vi "sendPriorityData.vi"(8 "error in (no error)":errorcluster, 9 "Additional content":string, 10 "Priority message":T1=enum."SetOffset", 11 "SM1000-control in":T2) -> (0 "error out":errorcluster, 3 "SM1000-control out":T2)   [LabVIEW 2013, in "SLMControl.lvlib" / "SM1000.lvclass"]
doc: "Send priority data to an EC device session.\n\nAn independent and parallel communication channel is provided to the controller to pass \"out-of-band\" commands. This channel of communication is used to send urgent commands to the controller, such as an abort message, or pause/resume messages.\nThe method returns as soon as the message is sent, not when the operation is actually performed on the target. Some messages, however, create response events when the action is completed, such as \"Abort\" or \"GetRegisters\"."
uses:
  SM1000.lvclass
  Object-reference.ctl
  Priority-messages.ctl
  SM1000.lvclass/SM1000.ctl
  Custom-errors.ctl
  C:/Users/vangeste/Desktop/2015-06-02 - SLM - MAIF/HC-HardwareCharacterization/Sources/SM1000/LECSession.dll
  HC-HardwareCharacterization/Sources/SM1000/LECSession.dll
  DOTNET-error-int.vi
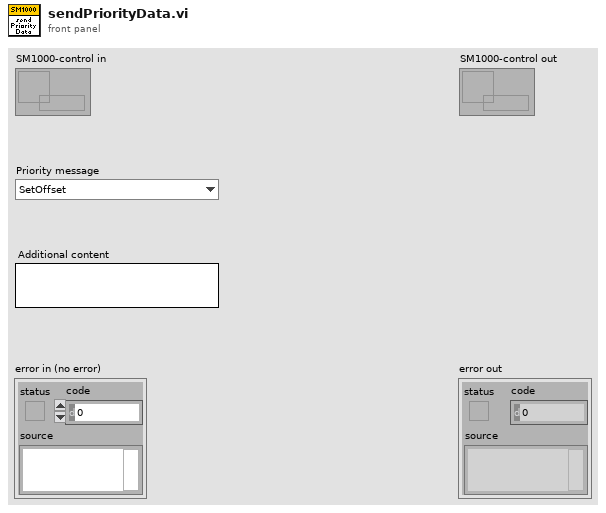
[diagram p1: front panel]
types:
  T1 = typedef "SLMControl.lvlib/SM1000.lvclass/Priority-messages.ctl" = enum16{"Abort", "Restart", "Suspend", "Resume", "GetRegisters", "SetInterlockEnable", "SetOffset"}
  T2 = typedef "SLMControl.lvlib/SM1000.lvclass/Object-reference.ctl" = refnum<data-value>
  T3 = typedef "SLMControl.lvlib/SM1000.lvclass/Custom-errors.ctl" = enum16{"No error", "Not implemented", "Command not recognized", "Invalid input", "No connection", "Timeout", "Resource not loaded"}
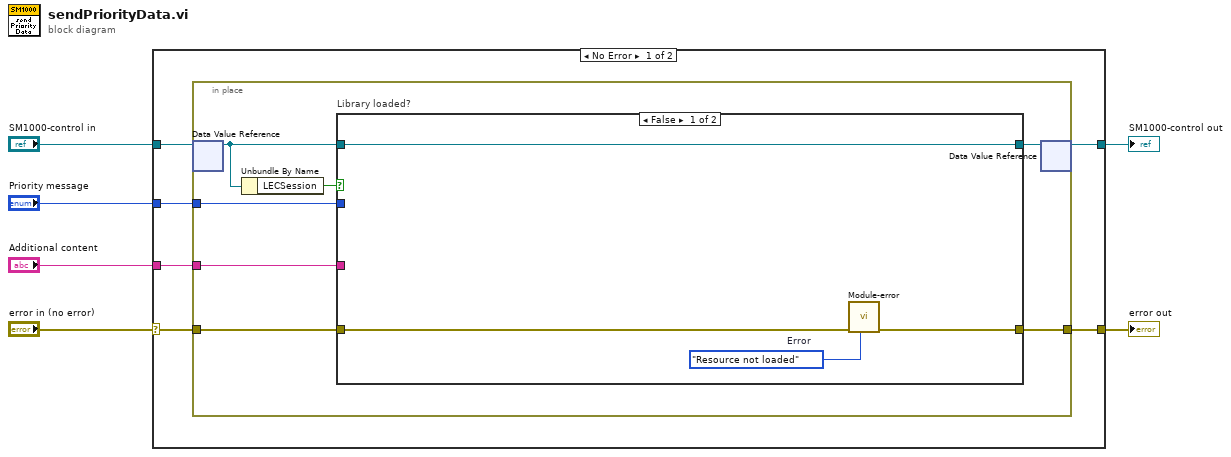
[diagram p0: block diagram]
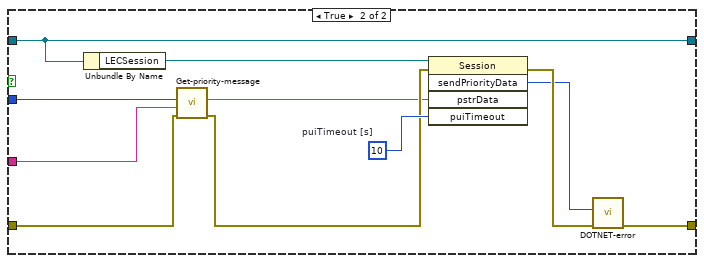
[diagram p2: hidden frame]
diagram:
  n1 = case shown="No Error" "error in (no error)" {
    selector: "error in (no error)" -> [w10 w36]
    tunnel: [w9 w36] -> w5
    tunnel: [w11 w35] -> w3
    tunnel: "SM1000-control in" -> [w12 w35]
    tunnel: "Priority message" -> [w8 _]
    tunnel: "Additional content" -> [w7 _]
    frame No Error {
      n2 = in-place {
        in-place-border: w10 -> [w19]
        in-place-border: [w16] -> w9
        in-place-border: w8 -> [w14]
        in-place-border: w7 -> [w13]
        n3 = in-place-dvr #1(w12) -> (w17:refnum<class "SM1000.lvclass">)  [unwired: 1 out]
        n4 = Unbundle By Name(w17) -> ("LECSession"=w18:bool)
        n5 = case "Library loaded?" shown="False" w18 {
          tunnel: w19 -> [w23 w29]
          tunnel: w17 -> [w21 w33]
          tunnel: [w22 w26] -> w16
          tunnel: [w21 w33] -> w15
          tunnel: w14 -> [_ w31]
          tunnel: w13 -> [_ w30]
          frame False {
            w20 = Custom-errors."Resource not loaded"  # Error
            n6 = call "Module-error.vi"("Error"=w20, "error in (no error)"=w23) -> ("error out"=w22:errorcluster)  [unwired: 9 in]
          }
          frame True {
            w32 = u32 10  # puiTimeout [s]
            n7 = Unbundle By Name(w33) -> ("LECSession"=w34:refnum<k24>)
            n8 = call "Get-priority-message.vi"("error in (no error)"=w29, "Additional content"=w30, "Priority message"=w31) -> ("error out"=w28:errorcluster, "Message string"=w27:string)  [unwired: 7 in]
            n9 = invoke class="Session" method="sendPriorityData"(reference=w34, error in=w28, "pstrData"=w27, "puiTimeout"=w32) -> (error out=w25:errorcluster, "sendPriorityData"=w24:u32)  [unwired: 1 in, 3 out]
            n10 = call-poly "DOTNET-error.vi"("error in (no error)"=w25, "Retun code"=w24) -> ("error out"=w26:errorcluster)  [unwired: 9 in]
          }
        }
        n11 = in-place-dvr #1(w15) -> (w11:T2)  [unwired: 1 out]
      }
    }
    frame Error {
    }
  }
  "error out" <- w5
  "SM1000-control out" <- w3
